vi "Tx_current_meas_postprocessing.vi"(0 "Original Waveform":waveform(dbl)(graph), 5 "cutoff pts length":i32, 7 "cutoff pts start index":i32, 9 "current sense scaling factor (mV/A)":dbl=40.0 format="%#_13g", 11 "desired frequency":dbl=25000.0 format="%#_13g", 12 "window":T1=1 items=["Rectangle"=0, "Hanning"=1, "Hamming"=2, "Blackman-Harris"=3, "Exact Blackman"=4, "Blackman"=5, "Flat Top"=6, "4 Term B-Harris "=7, "7 Term B-Harris"=8, "Low Sidelobe"=9, "Blackman Nuttall"=11, "Triangle"=30, "Bartlett-Hanning"=31, "Bohman"=32, "Parzen"=33, "Welch"=34, "Kaiser"=60, "Dolph-Chebyshev"=61, "Gaussian"=62]) -> (1 "f0-f9Mag":dbl[](array[numeric]), 2 "f0-f9Phase":dbl[](array[numeric]), 3 "THD":dbl format="%.2p", 4 "magnitude (Apk)":dbl, 6 "output phase":dbl, 8 "actual frequency selected":dbl, 10 "Tx current minmax array (A)":dbl[](array[numeric])=[0.5476160093058402, -0.45476671992115136], 14 "Hall DC (V)":dbl, 15 "AC rms (A)":dbl)   [LabVIEW 2021]
uses:
  <vilib>/Analysis/4window.llb/windowTd.ctl
  <vilib>/measure/matone.llb/Harmonic Distortion Analyzer 1 Chan.vi
  <vilib>/measure/maspectr.llb/FFT Spectrum (Mag-Phase) for 1 Chan.vi
  Human_Labview/global_variables.vi
  <vilib>/measure/NI_MAPro.lvlib
  <vilib>/Analysis/NI_AALPro.lvlib
panel:
  out "TX current meas":waveform(dbl)(graph)={"t0"=timestamp(3704229085.246047 s since 1904-01-01), "dt"=9.9999999999997e-07, "Y"=array[4000 elements], "attributes"=variant("NI_ChannelName"=variant(string "DAQ1/ai1"), "NI_UnitDescription"=variant(string "Volts"))}
  # "OUTPUTS:"
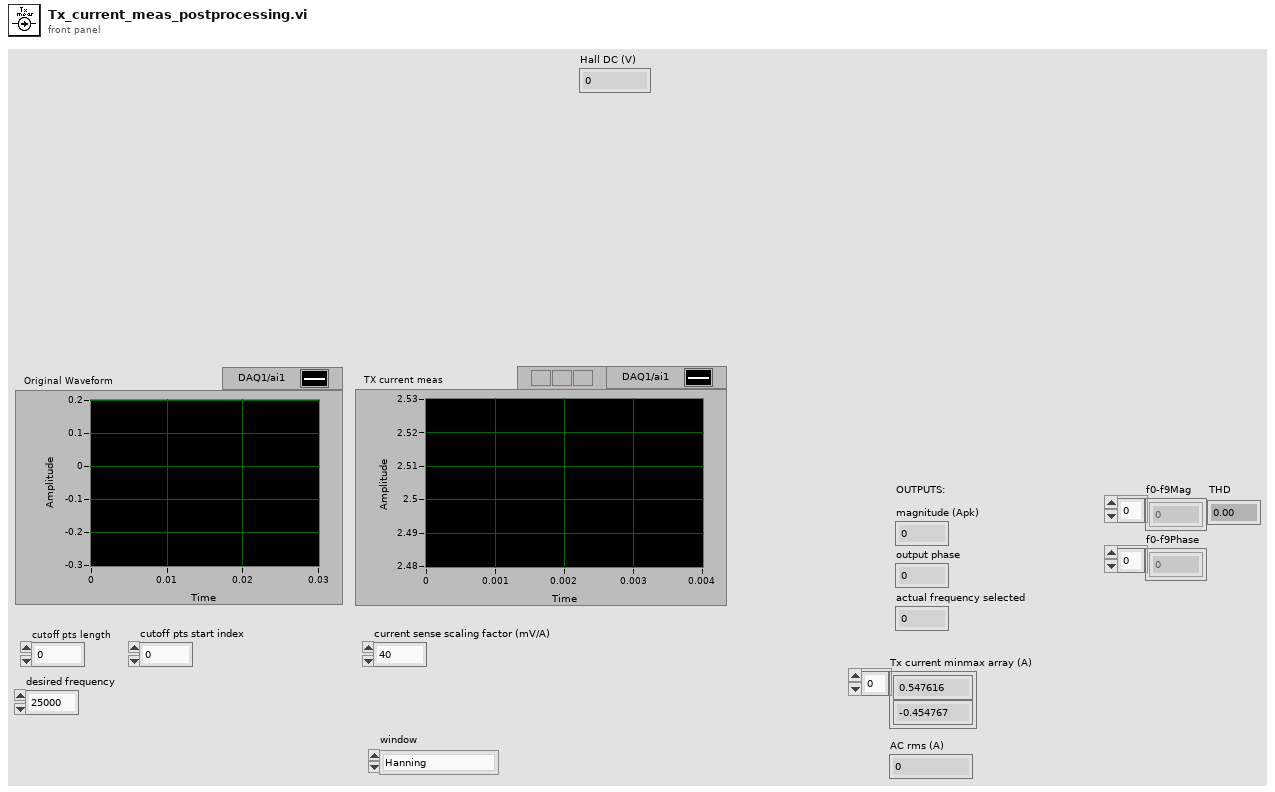
[diagram p1: front panel]
types:
  T1 = typedef "NI_AALPro.lvlib/windowTd.ctl" = u32
  T2 = cluster{"sample rate":dbl, "Transmit frequency":dbl, "Transmit amplitude":dbl, "sample rate digital out":dbl, "TX cycles":i32, "sample rate DAQ1":dbl, "Receive frequency":dbl, "Receive range":dbl, "TX harmonics":dbl[]}
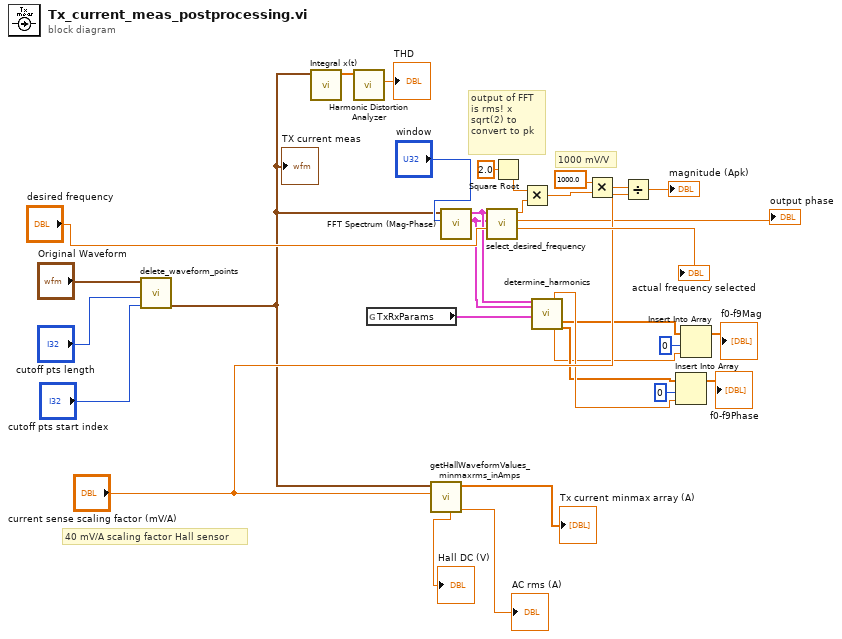
[diagram p0: block diagram]
diagram:
  # "40 mV/A scaling factor Hall sensor"
  # "output of FFT is rms! x sqrt(2) to convert to pk"
  # "1000 mV/V"
  n1 = call "delete_waveform_points.vi"("index"="cutoff pts start index", "length"="cutoff pts length", "Original Waveform"="Original Waveform") -> ("New Waveform"=w3:waveform(dbl))  [unwired: 8 in]
  "TX current meas" <- w3
  n2 = call <vilib>:"Integral x(t).vi"("X"=w3) -> ("Integral X"=w2:dbl[])  [unwired: 9 in, 1 out]
  n3 = call-poly <vilib>:"Harmonic Distortion Analyzer.vi"("signal in"=w2) -> ("THD"=→"THD":dbl)  [unwired: 5 in, 5 out]
  n4 = global read "global_variables.vi" "TxRxParams"() -> (w12:T2)
  n5 = call "getHallWaveformValues_minmaxrms_inAmps.vi"("waveform in"=w3, "Hall current sense scaling factor (mV/A)"="current sense scaling factor (mV/A)") -> ("DC (V)"=→"Hall DC (V)":dbl, "minmax array (A)"=→"Tx current minmax array (A)":dbl[], "AC rms (A)"=→"AC rms (A)":dbl)  [unwired: 4 in, 2 out]
  n6 = call-poly <vilib>:"FFT Spectrum (Mag-Phase).vi"("window"="window", "time signal"=w3) -> ("phase"=w13:cluster{"f0":dbl, "df":dbl, "phase":dbl[]}, "magnitude"=w14:cluster{"f0":dbl, "df":dbl, "magnitude":dbl[]})  [unwired: 5 in, 3 out]
  n7 = call "select_desired_frequency.vi"("desired frequency"="desired frequency", "FFT phase"=w13, "FFT magnitude"=w14) -> ("actual frequency selected"=→"actual frequency selected":dbl, "output phase"=→"output phase":dbl, "output magnitude"=w22:dbl)  [unwired: 6 in]
  n8 = Square Root(x=2.0) -> (sqrt(x)=w20:dbl)
  n9 = Multiply(x=w20, y=w22) -> (x*y=w21:dbl)
  n10 = call "determine_harmonics.vi"("FFT magnitude"=w14, "FFT phase"=w13, "TxRxParams"=w12) -> ("f0 phase"=w9:dbl, "f0 mag"=w4:dbl, "mag f2-f9"=w5:dbl[], "phase f2-f9"=w8:dbl[])  [unwired: 10 in, 3 out]
  n11 = Multiply(x=1000.0, y=w21) -> (x*y=w31:dbl)
  n12 = Divide(x=w31, y="current sense scaling factor (mV/A)") -> (x/y=→"magnitude (Apk)":dbl)
  n13 = Insert Into Array(array=w8, index=0, new element=w9) -> (→"f0-f9Phase":dbl[])
  n14 = Insert Into Array(array=w5, index=0, new element=w4) -> (→"f0-f9Mag":dbl[])
